vi "Autonomous Independent.vi"   [LabVIEW 2015]
doc: "This VI is called when autonomous begins, and will automatically be terminated when autonomous ends. You can carry out timed or sensor driven robot movement independently without needing to return to the caller."
uses:
  <vilib>/Rock Robotics/Network Tables/NT Read String.vi
  <vilib>/Rock Robotics/WPI/Utilities/WPI_GetSetVariantRefNum.vi
  <vilib>/Rock Robotics/Network Tables/NT Read Number.vi
  Robot Global Data.vi
types:
  T1 = typedef "WPI_RobotDriveDevRef.ctl" = cluster{"DevStatus":errorcluster, "Motors[]":T2[], "Square Inputs":bool, "Max Output":dbl}
  T2 = typedef "WPI_MotorControlDeviceRef.ctl" = cluster{"DeviceStatus":errorcluster, "Type":T3, "PWM":cluster{"PWM Channel":T4, "DeadBand":T5}, "CAN":cluster{"Device Number":u8, "Control Mode":T6, "Semaphore":T7, "Max Vout":dbl, "TalonSRX Control Mode":T8}, "Invert":bool}
  T3 = typedef "WPI_MotorControlType.ctl" = enum16{"PWM", "CAN", "CANTalonSRX"}
  T4 = typedef "FPGA_DIOPWMChannel.ctl" = enum8{"PWM 0", "PWM 1", "PWM 2", "PWM 3", "PWM 4", "PWM 5", "PWM 6", "PWM 7", "PWM 8", "PWM 9", "PWM MXP 0", "PWM MXP 1", "PWM MXP 2", "PWM MXP 3", "PWM MXP 4", "PWM MXP 5", "PWM MXP 6", "PWM MXP 7", "PWM MXP 8", "PWM MXP 9", "Invalid"}
  T5 = typedef "WPI_PWMDeadband.ctl" = cluster{"Name":string, "maxPositivePwm":i32, "minPositivePwm":i32, "centerPwm":i32, "maxNegativePwm":i32, "minNegativePwm":i32, "angularRange":u16}
  T6 = typedef "WPI_CANJaguar_ControlMode.ctl" = enum8{"Percent VBus", "Current", "Speed", "Position", "Voltage"}
  T7 = typedef "Semaphore RefNum" = refnum<k1>
  T8 = typedef "WPI_CANTalonSRX_APIControlMode.ctl" = enum8{"Percent VBus", "Speed", "Position", "Slave", "Unchanged / Invalid", "Voltage Compensation", "Current", "Motion Profile"}
  T9 = enum8{"Low Bar", "Porticullis", "Cheval de Frise", "Moat", "Ramparts", "Drawbridge", "Sally Port", "Rock Wall", "Rough Terrain"}
  T10 = enum16{"First Run", "Initial Angle", "Driving", "Final Angle", "Done"}
  T11 = cluster{"Mode":enum16{"First Run", "Initial Angle", "Driving", "Final Angle", "Done"}, "Calc. Tgt. Angle":dbl, "Backwards?":bool}
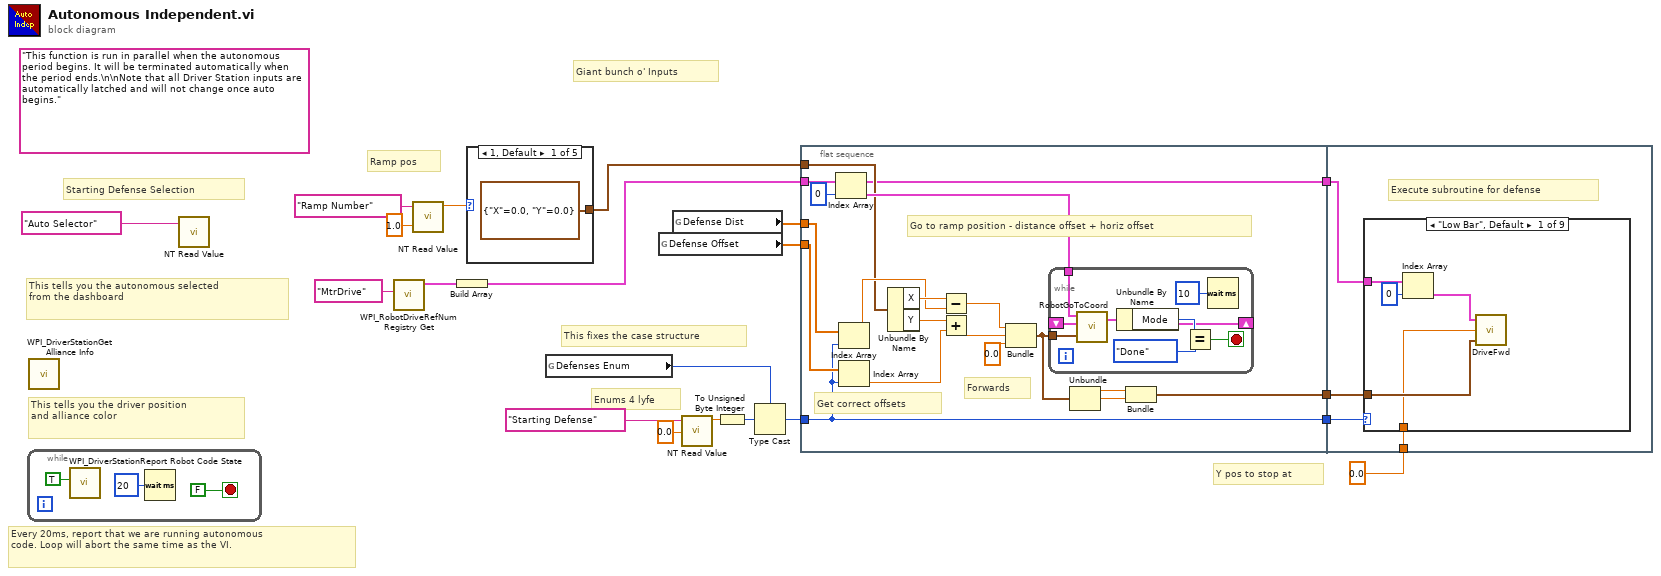
[diagram p0: block diagram]
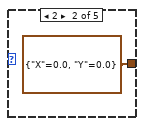
[diagram p2: hidden frame]
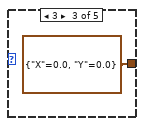
[diagram p3: hidden frame]
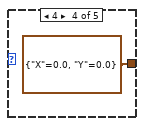
[diagram p4: hidden frame]
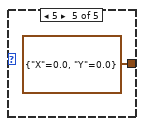
[diagram p5: hidden frame]
diagram:
  (unwired) "This function is run in parallel when the autonomous period begins. It will be terminated automatically when the period ends.\n\nNote that all Driver Station inputs are automatically latched and will not change once auto begins."
  # "Y pos to stop at"
  # "Ramp pos"
  # "Giant bunch o' Inputs"
  # "This fixes the case structure"
  # "Enums 4 lyfe"
  # "Starting Defense Selection"
  # "This tells you the autonomous selected\nfrom the dashboard"
  # "Every 20ms, report that we are running autonomous\ncode. Loop will abort the same time as the VI."
  # "This tells you the driver position\nand alliance color"
  n1 = while {
    stop <- FALSE stop-if-true
    n2 = call <vilib>:"WPI_DriverStationReport Robot Code State.vi"("Autonomous"=TRUE) -> ()  [unwired: 10 in, 1 out]
    n3 = Wait (ms)(milliseconds to wait=u32 20) -> ()  [unwired: 1 out]
  }
  n4 = call <vilib>:"WPI_DriverStationGet Alliance Info.vi"() -> ()  [unwired: 12 out]
  n5 = call-poly <vilib>:"NT Read Value.vi"("Name"="Auto Selector") -> ()  [unwired: 9 in, 2 out]
  n6 = call <vilib>:"WPI_RobotDriveRefNum Registry Get.vi"("refnum name"="MtrDrive") -> ("RobotDriveDevRef"=w5:T1)  [unwired: 9 in, 1 out]
  n7 = call-poly <vilib>:"NT Read Value.vi"("Default Value"=1.0, "Name"="Ramp Number") -> ("Numeric"=w8:dbl)  [unwired: 8 in, 1 out]
  n8 = Build Array(w5) -> (w4:T1[])
  n9 = case shown="1, Default" w8 {
    tunnel: [cluster{"X":dbl, "Y":dbl} {"X"=0.0, "Y"=0.0} cluster{"X":dbl, "Y":dbl} {"X"=0.0, "Y"=0.0} cluster{"X":dbl, "Y":dbl} {"X"=0.0, "Y"=0.0} cluster{"X":dbl, "Y":dbl} {"X"=0.0, "Y"=0.0} cluster{"X":dbl, "Y":dbl} {"X"=0.0, "Y"=0.0}] -> w6
    frame 1, Default {
    }
    frame 2 {
    }
    frame 3 {
    }
    frame 4 {
    }
    frame 5 {
    }
  }
  n10 = global read "Robot Global Data.vi" "Defenses Enum"() -> (w15:T9)
  n11 = global read "Robot Global Data.vi" "Defense Offset"() -> (w10:dbl[])
  n12 = global read "Robot Global Data.vi" "Defense Dist"() -> (w11:dbl[])
  n13 = call-poly <vilib>:"NT Read Value.vi"("Default Value"=0.0, "Name"="Starting Defense") -> ("Numeric"=w18:dbl)  [unwired: 8 in, 1 out]
  n14 = To Unsigned Byte Integer(number=w18) -> (unsigned 8bit integer=w17:u8)
  n15 = Type Cast(type=w15, x=w17) -> (*(type *) &x=w16:T9)
  n16 = flat-sequence {
    tunnel: w16 -> [w41]
    tunnel: [w41] -> w14
    tunnel: w4 -> [w33]
    tunnel: w11 -> [w43]
    tunnel: w10 -> [w42]
    tunnel: w6 -> [w34]
    tunnel: [w33] -> w3
    tunnel: [w29] -> w2
    tunnel: w14 -> [w58]
    tunnel: w3 -> [w57]
    tunnel: w2 -> [w56]
    tunnel: 0.0 -> [w55]
    frame #0 {
      # "Get correct offsets"
      # "Forwards"
      # "Go to ramp position - distance offset + horiz offset"
      n17 = Index Array(array=w33, index=0) -> (element=w44:T1)
      n18 = Index Array(array=w43, index=w41) -> (element=w35:dbl)
      n19 = Index Array(array=w42, index=w41) -> (element=w39:dbl)
      n20 = Unbundle By Name(w34) -> ("X"=w36:dbl, "Y"=w40:dbl)
      n21 = Subtract(x=w36, y=w35) -> (x-y=w37:dbl)
      n22 = Add(x=w40, y=w39) -> (x+y=w38:dbl)
      n23 = Bundle(w37, w38, 0.0) -> (w32:cluster{dbl, dbl, dbl})  [unwired: 1 in]
      n24 = while {
        tunnel: w44 -> [w54]
        shift-right: [w50] -> _
        shift-left: _ -> [w49]
        tunnel: w32 -> [w48]
        stop <- w51 stop-if-true
        n25 = call "RobotGoToCoord.vi"("X/Y/a Target"=w48, "Status Input"=w49, "RobotDriveDevRef"=w54) -> ("Status Output"=w50:T11)  [unwired: 1 in, 1 out]
        n26 = Unbundle By Name(w50) -> ("Mode"=w53:T10)
        n27 = Equal?(x=w53, y=T10."Done") -> (x = y?=w51:bool)
        n28 = Wait (ms)(milliseconds to wait=u32 10) -> ()  [unwired: 1 out]
      }
      n29 = Unbundle(w32) -> (w31:dbl, w30:dbl)  [unwired: 1 out]
      n30 = Bundle(w31, w30) -> (w29:cluster{dbl, dbl})  [unwired: 1 in]
    }
    frame #1 {
      # "Execute subroutine for defense"
      n31 = case shown="\"Low Bar\", Default" w58 {
        tunnel: w57 -> [w63 _ _ _ _ _ _ _ _]
        tunnel: w56 -> [w60 _ _ _ _ _ _ _ _]
        tunnel: w55 -> [w59 _ _ _ _ _ _ _ _]
        frame "Low Bar", Default {
          n32 = Index Array(array=w63, index=0) -> (element=w61:T1)
          n33 = call "DriveFwd.vi"("Start X/Y"=w60, "Stop Y Pos"=w59, "DriveRef"=w61) -> ()  [unwired: 1 in]
        }
        frame "Porticullis" {
        }
        frame "Cheval de Frise" {
        }
        frame "Moat" {
        }
        frame "Ramparts" {
        }
        frame "Drawbridge" {
        }
        frame "Sally Port" {
        }
        frame "Rock Wall" {
        }
        frame "Rough Terrain" {
        }
      }
    }
  }
